vi "SetControlValueHTTP.vi"(5 "silent (false)":bool, 7 "Service":string="http://127.0.0.1/labview", 8 "error in":errorcluster, 9 "value":string, 10 "ctrl":string, 11 "vi":string) -> (0 "error out":errorcluster, 1 "value":string)   [LabVIEW 2020]
uses:
  <vilib>/httpClient/LabVIEWHTTPClient.lvlib
  <vilib>/wsapi/NI_WebServices.lvlib
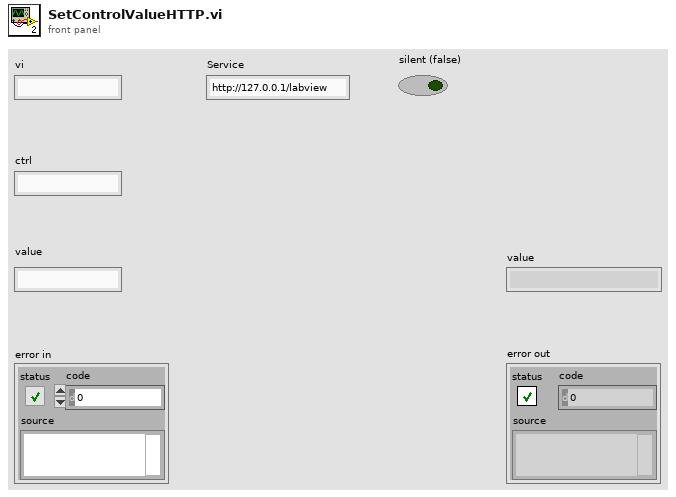
[diagram p1: front panel]
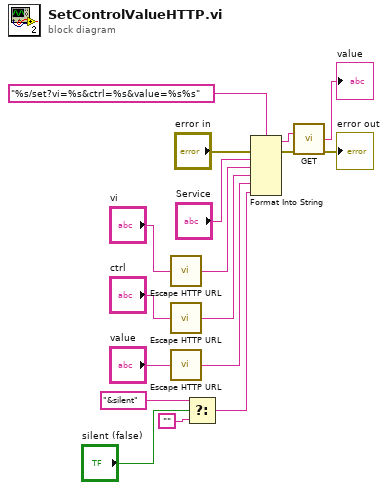
[diagram p0: block diagram]
diagram:
  n1 = call <vilib>:"Escape HTTP URL.vi"("unescaped string in"="vi") -> ("escaped string out"=w11:string)
  n2 = call <vilib>:"Escape HTTP URL.vi"("unescaped string in"="ctrl") -> ("escaped string out"=w9:string)
  n3 = call <vilib>:"Escape HTTP URL.vi"("unescaped string in"="value") -> ("escaped string out"=w1:string)
  n4 = Select(t="&silent", s="silent (false)", f="") -> (s? t:f=w2:string)
  n5 = Format Into String(format string="%s/set?vi=%s&ctrl=%s&value=%s%s", error in="error in", "Service", w11, w9, w1, w2) -> (resulting string=w8:string, error out=w5:errorcluster)  [unwired: 1 in]
  n6 = call <vilib>:"GET.vi"("url"=w8, "error in (no error)"=w5) -> ("body"=→"value":string, "error out"=→"error out":errorcluster)  [unwired: 10 in, 2 out]
